vi "Number to Multiplex.vi"(1 "Numeric":u32) -> (0 "Start-Stop1 Multyplex 2":T1)   [LabVIEW 2012]
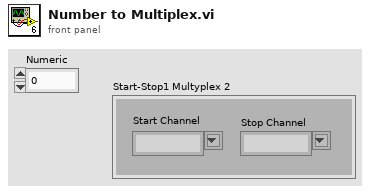
[diagram p1: front panel]
types:
  T1 = cluster{"Start Channel":string, "Stop Channel":string}
  T2 = cluster{"Boolean array[0]":bool, "Boolean array[1]":bool, "Boolean array[2]":bool, "Boolean array[3]":bool, "Boolean array[4]":bool, "Boolean array[5]":bool, "Boolean array[6]":bool, "Boolean array[7]":bool, "Boolean array[8]":bool}
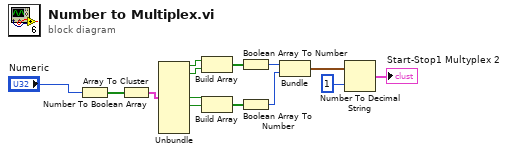
[diagram p0: block diagram]
diagram:
  n1 = Number To Boolean Array(number="Numeric") -> (Boolean array=w13:bool[])
  n2 = Array To Cluster(array=w13) -> (cluster=w5:T2)
  n3 = Unbundle(w5) -> ("Boolean array[0]"=w4:bool, "Boolean array[1]"=w3:bool, "Boolean array[4]"=w2:bool, "Boolean array[5]"=w1:bool)  [unwired: 5 out]
  n4 = Build Array(w4, w3) -> (w12:bool[])
  n5 = Build Array(w2, w1) -> (w11:bool[])
  n6 = Boolean Array To Number(Boolean array=w12) -> (number=w10:u32)
  n7 = Boolean Array To Number(Boolean array=w11) -> (number=w9:u32)
  n8 = Bundle(w10, w9) -> (w8:cluster{u32, u32})  [unwired: 1 in]
  n9 = Number To Decimal String(number=w8, width (-)=i16 1) -> (decimal integer string=→"Start-Stop1 Multyplex 2":cluster{string, string})
